vi "HIOKI PW3390 VI_Tree.vi"   [LabVIEW 2009]
uses:
  <instrlib>/PW3390/Common/_Initialize/HIOKI PW3390 Initialize LAN.vi
  <instrlib>/PW3390/Configure/Motor/_CH A/HIOKI PW3390 Conf CH A DC.vi
  <instrlib>/PW3390/Configure/Motor/_CH B/HIOKI PW3390 Conf CH B Pulse.vi
panel:
  # "SEE DIAGRAM\nFOR VI TREE."
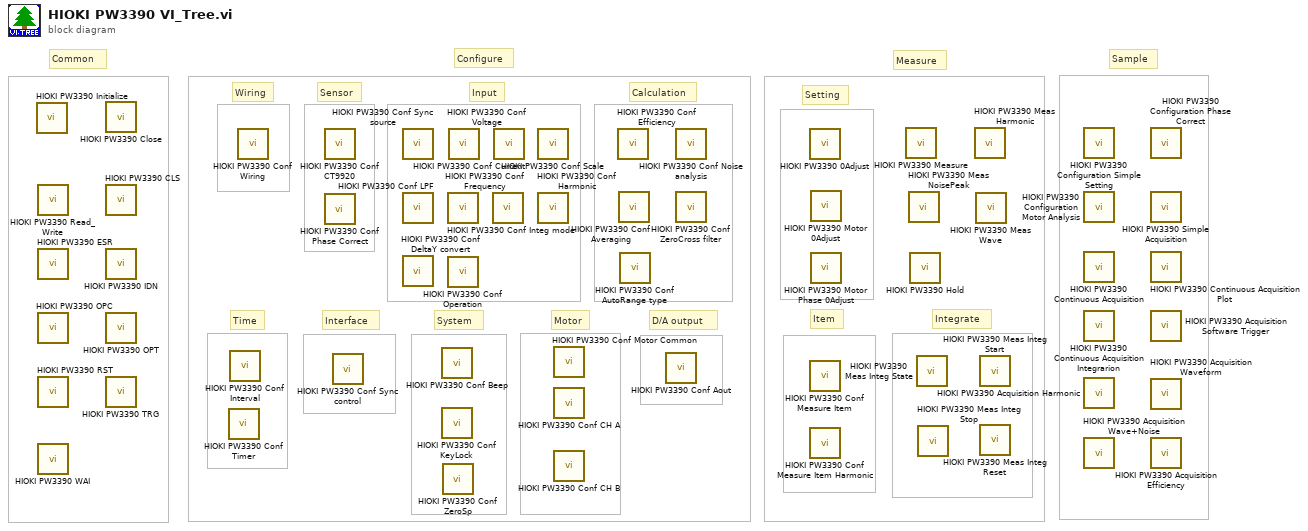
[diagram p0: block diagram]
diagram:
  # "Integrate"
  # "Item"
  # "Setting"
  # "D/A output"
  # "Motor"
  # "System"
  # "Interface"
  # "Time"
  # "Calculation"
  # "Input"
  # "Sensor"
  # "Wiring"
  # "Sample"
  # "Measure"
  # "Configure"
  # "Common"
  n1 = call-poly <instrlib>:"HIOKI PW3390 Initialize.vi"() -> ()  [unwired: 13 in, 3 out]
  n2 = call <instrlib>:"HIOKI PW3390 Read_Write.vi"() -> ()  [unwired: 9 in, 3 out]
  n3 = call <instrlib>:"HIOKI PW3390 ESR.vi"() -> ()  [unwired: 8 in, 4 out]
  n4 = call <instrlib>:"HIOKI PW3390 OPC.vi"() -> ()  [unwired: 9 in, 3 out]
  n5 = call <instrlib>:"HIOKI PW3390 RST.vi"() -> ()  [unwired: 10 in, 2 out]
  n6 = call <instrlib>:"HIOKI PW3390 WAI.vi"() -> ()  [unwired: 10 in, 2 out]
  n7 = call <instrlib>:"HIOKI PW3390 Close.vi"() -> ()  [unwired: 15 in, 1 out]
  n8 = call <instrlib>:"HIOKI PW3390 CLS.vi"() -> ()  [unwired: 10 in, 2 out]
  n9 = call <instrlib>:"HIOKI PW3390 IDN.vi"() -> ()  [unwired: 9 in, 3 out]
  n10 = call <instrlib>:"HIOKI PW3390 OPT.vi"() -> ()  [unwired: 9 in, 3 out]
  n11 = call <instrlib>:"HIOKI PW3390 TRG.vi"() -> ()  [unwired: 10 in, 2 out]
  n12 = call <instrlib>:"HIOKI PW3390 Conf Timer.vi"() -> ()  [unwired: 12 in, 4 out]
  n13 = call <instrlib>:"HIOKI PW3390 Conf Interval.vi"() -> ()  [unwired: 13 in, 3 out]
  n14 = call <instrlib>:"HIOKI PW3390 Conf Wiring.vi"() -> ()  [unwired: 13 in, 3 out]
  n15 = call <instrlib>:"HIOKI PW3390 Conf CT9920.vi"() -> ()  [unwired: 13 in, 3 out]
  n16 = call <instrlib>:"HIOKI PW3390 Conf Phase Correct.vi"() -> ()  [unwired: 11 in, 5 out]
  n17 = call <instrlib>:"HIOKI PW3390 Conf Sync control.vi"() -> ()  [unwired: 12 in, 4 out]
  n18 = call <instrlib>:"HIOKI PW3390 Conf Sync source.vi"() -> ()  [unwired: 13 in, 3 out]
  n19 = call <instrlib>:"HIOKI PW3390 Conf LPF.vi"() -> ()  [unwired: 13 in, 3 out]
  n20 = call <instrlib>:"HIOKI PW3390 Conf DeltaY convert.vi"() -> ()  [unwired: 13 in, 3 out]
  n21 = call <instrlib>:"HIOKI PW3390 Conf Beep.vi"() -> ()  [unwired: 9 in, 3 out]
  n22 = call <instrlib>:"HIOKI PW3390 Conf KeyLock.vi"() -> ()  [unwired: 13 in, 3 out]
  n23 = call <instrlib>:"HIOKI PW3390 Conf ZeroSp.vi"() -> ()  [unwired: 13 in, 3 out]
  n24 = call <instrlib>:"HIOKI PW3390 Conf Integ mode.vi"() -> ()  [unwired: 13 in, 3 out]
  n25 = call <instrlib>:"HIOKI PW3390 Conf Operation.vi"() -> ()  [unwired: 13 in, 3 out]
  n26 = call <instrlib>:"HIOKI PW3390 Conf Voltage.vi"() -> ()  [unwired: 11 in, 5 out]
  n27 = call <instrlib>:"HIOKI PW3390 Conf Frequency.vi"() -> ()  [unwired: 12 in, 4 out]
  n28 = call <instrlib>:"HIOKI PW3390 Conf Current.vi"() -> ()  [unwired: 11 in, 5 out]
  n29 = call <instrlib>:"HIOKI PW3390 Conf Scale.vi"() -> ()  [unwired: 12 in, 4 out]
  n30 = call <instrlib>:"HIOKI PW3390 Conf Harmonic.vi"() -> ()  [unwired: 12 in, 4 out]
  n31 = call <instrlib>:"HIOKI PW3390 Conf Motor Common.vi"() -> ()  [unwired: 11 in, 5 out]
  n32 = call-poly <instrlib>:"HIOKI PW3390 Conf CH A.vi"() -> ()  [unwired: 10 in, 6 out]
  n33 = call-poly <instrlib>:"HIOKI PW3390 Conf CH B.vi"() -> ()  [unwired: 12 in, 8 out]
  n34 = call <instrlib>:"HIOKI PW3390 Conf Efficiency.vi"() -> ()  [unwired: 12 in, 4 out]
  n35 = call <instrlib>:"HIOKI PW3390 Conf Averaging.vi"() -> ()  [unwired: 13 in, 3 out]
  n36 = call <instrlib>:"HIOKI PW3390 Conf AutoRange type.vi"() -> ()  [unwired: 13 in, 3 out]
  n37 = call <instrlib>:"HIOKI PW3390 Conf Aout.vi"() -> ()  [unwired: 13 in, 7 out]
  n38 = call <instrlib>:"HIOKI PW3390 Conf Noise analysis.vi"() -> ()  [unwired: 13 in, 7 out]
  n39 = call <instrlib>:"HIOKI PW3390 Conf ZeroCross filter.vi"() -> ()  [unwired: 13 in, 3 out]
  n40 = call <instrlib>:"HIOKI PW3390 0Adjust.vi"() -> ()  [unwired: 13 in, 3 out]
  n41 = call <instrlib>:"HIOKI PW3390 Conf Measure Item.vi"() -> ()  [unwired: 19 in, 9 out]
  n42 = call <instrlib>:"HIOKI PW3390 Conf Measure Item Harmonic.vi"() -> ()  [unwired: 14 in, 6 out]
  n43 = call <instrlib>:"HIOKI PW3390 Motor 0Adjust.vi"() -> ()  [unwired: 14 in, 2 out]
  n44 = call <instrlib>:"HIOKI PW3390 Motor Phase 0Adjust.vi"() -> ()  [unwired: 14 in, 2 out]
  n45 = call <instrlib>:"HIOKI PW3390 Measure.vi"() -> ()  [unwired: 10 in, 6 out]
  n46 = call <instrlib>:"HIOKI PW3390 Meas NoisePeak.vi"() -> ()  [unwired: 10 in, 6 out]
  n47 = call <instrlib>:"HIOKI PW3390 Hold.vi"() -> ()  [unwired: 13 in, 3 out]
  n48 = call <instrlib>:"HIOKI PW3390 Meas Integ State.vi"() -> ()  [unwired: 13 in, 3 out]
  n49 = call <instrlib>:"HIOKI PW3390 Meas Integ Stop.vi"() -> ()  [unwired: 14 in, 2 out]
  n50 = call <instrlib>:"HIOKI PW3390 Meas Harmonic.vi"() -> ()  [unwired: 10 in, 6 out]
  n51 = call <instrlib>:"HIOKI PW3390 Meas Wave.vi"() -> ()  [unwired: 5 in, 11 out]
  n52 = call <instrlib>:"HIOKI PW3390 Meas Integ Start.vi"() -> ()  [unwired: 14 in, 2 out]
  n53 = call <instrlib>:"HIOKI PW3390 Meas Integ Reset.vi"() -> ()  [unwired: 14 in, 2 out]
  n54 = call <instrlib>:"HIOKI PW3390 Configuration Simple Setting.vi"() -> ()  [unwired: 1 in]
  n55 = call <instrlib>:"HIOKI PW3390 Configuration Motor Analysis.vi"() -> ()  [unwired: 1 in]
  n56 = call <instrlib>:"HIOKI PW3390 Continuous Acquisition.vi"() -> ()  [unwired: 1 in]
  n57 = call <instrlib>:"HIOKI PW3390 Continuous Acquisition Integrarion.vi"() -> ()  [unwired: 1 in]
  n58 = call <instrlib>:"HIOKI PW3390 Acquisition Harmonic.vi"() -> ()  [unwired: 12 in]
  n59 = call <instrlib>:"HIOKI PW3390 Acquisition Wave+Noise.vi"() -> ()  [unwired: 1 in]
  n60 = call <instrlib>:"HIOKI PW3390 Configuration Phase Correct.vi"() -> ()  [unwired: 1 in]
  n61 = call <instrlib>:"HIOKI PW3390 Simple Acquisition.vi"() -> ()  [unwired: 1 in]
  n62 = call <instrlib>:"HIOKI PW3390 Continuous Acquisition Plot.vi"() -> ()  [unwired: 1 in]
  n63 = call <instrlib>:"HIOKI PW3390 Acquisition Software Trigger.vi"() -> ()  [unwired: 1 in]
  n64 = call <instrlib>:"HIOKI PW3390 Acquisition Waveform.vi"() -> ()  [unwired: 1 in]
  n65 = call <instrlib>:"HIOKI PW3390 Acquisition Efficiency.vi"() -> ()  [unwired: 1 in]
